vi "RT_main.vi"() -> ()   [LabVIEW 2025]
uses:
  Game Data.ctl
  Bullet Data.ctl
  Game State.ctl
  <vilib>/FPGAPlugInAG/myRIO-1900/niLvFpga_Open_myRIO-1900.vi
  <vilib>/rvi/interface/common/dynamic/niFpgaDynamicAddResources.vi
  <vilib>/Utility/error.llb/Error Cluster From Error Code.vi
  <vilib>/rvi/errors/niLvFpgaAdjustHostInterfaceError.vi
  <vilib>/FPGAPlugInAG/Dynamic/niLvFpga_Close_Dynamic.vi
  <vilib>/rvi/interface/nirviOpenFPGA/nirviOpenFPGA.xnode
  FPGA Bitfiles/myledsnake_FPGATarget2_FPGAmain_jKt4U3oCCCU.lvbitx
  FPGA_main.vi
  <vilib>/rvi/interface/nirviReadWriteControl/nirviReadWriteControl.xnode
  <vilib>/rvi/interface/nirviMethod/nirviMethod.xnode
  <vilib>/rvi/interface/nirviCloseFPGA/nirviCloseFPGA.xnode
  <vilib>/FPGAPlugInAG/Dynamic/niLvFpga_WriteFifo_Dynamic.vi
  <vilib>/rvi/errors/niLvFpgaMergeErrorWithErrorCode.vi
  NiFpgaLv.dll
  <vilib>/rvi/interface/Simulation/niFpgaSimulationCallBeginRW.vi
panel:
  out "LEDs":u32[](array[colorbox])
  in  "Stop":bool
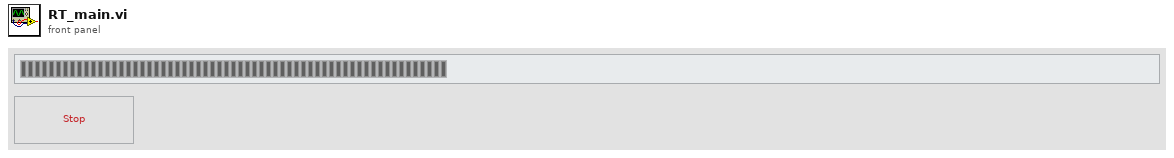
[diagram p1: front panel]
types:
  T1 = typedef "Game State.ctl" = enum16{"Reset", "Idle", "Start", "Playing", "Win", "Lose"}
  T2 = typedef "Game Data.ctl" = cluster{"Snake":u32[], "Snake Speed":dbl, "Pixels":u32[], "Bullet Speed":dbl, "Snake Position":dbl, "Bullets":T3[]}
  T3 = typedef "Bullet Data.ctl" = cluster{"position":dbl, "color":u32}
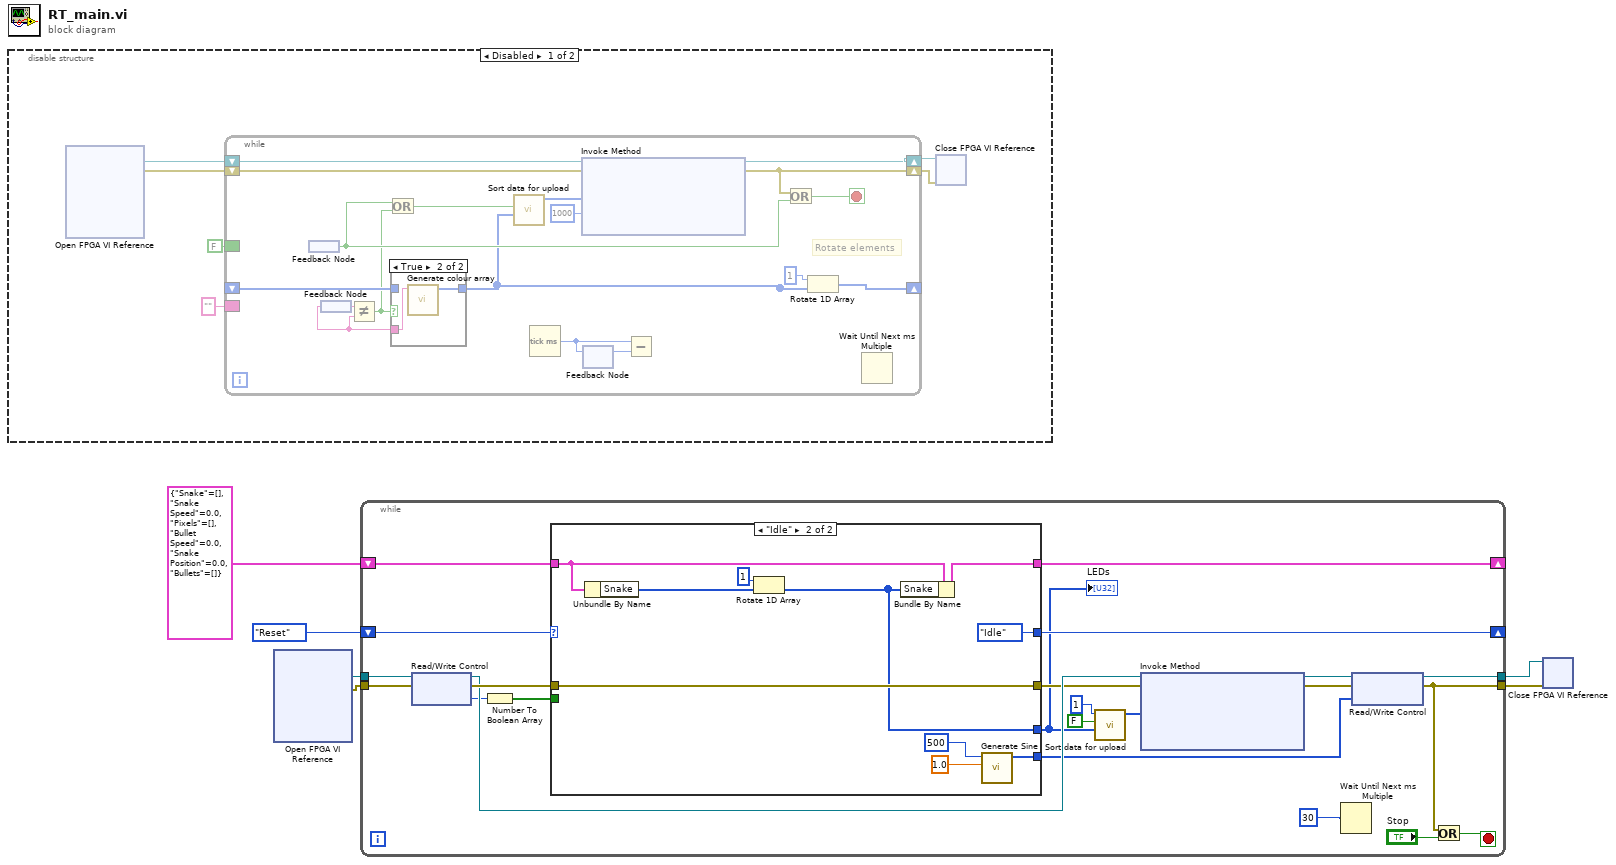
[diagram p0: block diagram]
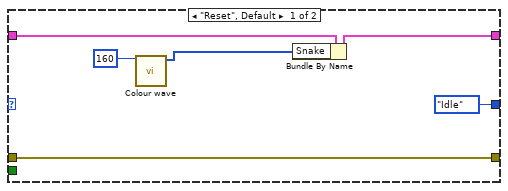
[diagram p2: hidden frame]
diagram:
  n1 = disable-structure shown="Disabled" {
    frame Disabled {
      n2 = xnode "Open FPGA VI Reference"() -> ("FPGA VI Reference Out"=w12:refnum<k20>, "error out"=w11:errorcluster)  [unwired: 2 in]
      n3 = while {
        shift-right: [w25] -> w9
        shift-left: w11 -> [w32]
        shift-right: [w33] -> w10
        shift-left: w12 -> [w31]
        shift-right: [w30] -> _
        shift-left: _ -> [w17]
        border: FALSE ("stop") -> [_]
        border: "" ("Pattern") -> [_]
        stop <- w26 stop-if-true
        # "Rotate elements"
        n4 = feedback-in #1() -> (w21:bool)
        n5 = feedback #1() -> (w20:bool)
        n6 = feedback #2() -> (w18:string)
        n7 = Not Equal?(x=w18) -> (y=w15:string, x != y?=w13:bool)
        n8 = feedback-in #2(w15) -> ()
        n9 = Or(x=w20, y=w13) -> (x .or. y?=w14:bool)
        n10 = case shown="True" w13 {
          tunnel: [w34 w36] -> w16
          tunnel: w17 -> [w34 _]
          tunnel: w15 -> [_ w35]
          frame False {
          }
          frame True {
            n11 = call "Generate colour array.vi"("Combo Box"=w35) -> ("Array"=w36:u32[])  [unwired: 10 in]
          }
        }
        n12 = call "Sort data for upload.vi"("Colour array in"=w16, "Zero Outputs?"=w14) -> ("Upload data"=w19:u32[])  [unwired: 9 in]
        n13 = Tick Count (ms)() -> (millisecond timer value=w23:u32)
        n14 = xnode "Invoke Method"("FPGA VI Reference In"=w31, "error in"=w32, "Data"=w19, "Timeout (ms)"=1000) -> ("FPGA VI Reference Out"=w33:refnum<k20>, "error out"=w25:errorcluster)  [unwired: 1 out]
        n15 = feedback-in #3(w23) -> ()
        n16 = feedback #3() -> (w24:u32)  [unwired: 1 in]
        n17 = Subtract(x=w23, y=w24) -> (x-y=w22:u32)
        n18 = Or(x=w25, y=w20) -> (x .or. y?=w26:bool)
        n19 = Rotate 1D Array(1:w16, 2:1 ("n")) -> (0:w30:u32[])
        n20 = Wait Until Next ms Multiple() -> (millisecond multiple=w27:u32)  [unwired: 1 out]
      }
      n21 = xnode "Close FPGA VI Reference"("FPGA VI Reference In"=w10, "error in"=w9) -> ()  [unwired: 1 out]
    }
    frame Enabled {
    }
  }
  n22 = xnode "Open FPGA VI Reference"() -> ("FPGA VI Reference Out"=w6:refnum<k20>, "error out"=w5:errorcluster)  [unwired: 2 in]
  n23 = while {
    tunnel: w6 -> [w56]
    tunnel: w5 -> [w59]
    tunnel: [w52] -> w4
    tunnel: [w38] -> w3
    shift-right: [w49] -> _
    shift-left: Game_State."Reset" -> [w50]
    shift-right: [w47] -> _
    shift-left: T2 {"Snake"=[], "Snake Speed"=0.0, "Pixels"=[], "Bullet Speed"=0.0, "Snake Position"=0.0, "Bullets"=[]} -> [w48]
    stop <- w39 stop-if-true
    n24 = xnode "Read/Write Control"("FPGA VI Reference In"=w56, "error in"=w59) -> ("FPGA VI Reference Out"=w55:refnum<k20>, "error out"=w57:errorcluster, "buttons"=w54:u64)
    n25 = Number To Boolean Array(number=w54) -> (Boolean array=w46:bool[])
    n26 = case shown="\"Idle\"" w50 {
      tunnel: w57 -> [w64 w75]
      tunnel: [w64 w75] -> w51
      tunnel: [Game_State."Idle" Game_State."Idle"] -> w49
      tunnel: [w62 w72] -> w47
      tunnel: w48 -> [w63 w73]
      tunnel: w46 -> [_ _]
      tunnel: [_ w69] -> w37
      tunnel: [_ w68] -> w42
      frame "Reset", Default {
        n27 = call "Colour wave.vi"("Numeric"=160) -> ("Array"=w60:u32[])  [unwired: 10 in]
        n28 = Bundle By Name(cluster=w63, "Snake"=w60) -> (w62:T2)
      }
      frame "Idle" {
        n29 = Unbundle By Name(w73) -> ("Snake"=w71:u32[])
        n30 = Rotate 1D Array(1:w71, 2:1 ("n")) -> (0:w69:u32[])
        n31 = Bundle By Name(cluster=w73, "Snake"=w69) -> (w72:T2)
        n32 = call "Generate Sine.vi"("brightness"=1.0, "period (ms)"=u32 500) -> ("sine"=w68:i32[])  [unwired: 9 in]
      }
    }
    "LEDs" <- w37
    n33 = call "Sort data for upload.vi"("Colour array in"=w37, "Zero Outputs?"=FALSE, "ID"=u32 1) -> ("Upload data"=w45:u32[])  [unwired: 8 in]
    n34 = xnode "Invoke Method"("FPGA VI Reference In"=w55, "error in"=w51, "Data"=w45) -> ("FPGA VI Reference Out"=w53:refnum<k20>, "error out"=w58:errorcluster)  [unwired: 1 in, 1 out]
    n35 = Wait Until Next ms Multiple(millisecond multiple=u32 30) -> ()  [unwired: 1 out]
    n36 = xnode "Read/Write Control"("FPGA VI Reference In"=w53, "error in"=w58, "hightimes"=w42) -> ("FPGA VI Reference Out"=w52:refnum<k20>, "error out"=w38:errorcluster)
    n37 = Or(x=w38, y="Stop") -> (x .or. y?=w39:bool)
  }
  n38 = xnode "Close FPGA VI Reference"("FPGA VI Reference In"=w4, "error in"=w3) -> ()  [unwired: 1 out]
